vi "init.vi"(8 "error in (no error)":errorcluster, 10 "Resource":string, 11 "ScopeNi in":refnum<class "ScopeNi.lvclass">) -> (0 "error out":errorcluster, 3 "ScopeNi out":refnum<class "ScopeNi.lvclass">)   [LabVIEW 2023, in "ScopeNi.lvclass"]
doc: "Initialize the instrument by a given resource string or alias name"
uses:
  ScopeNi.lvclass
  ScopeNi.lvclass/ScopeNi.ctl
  <instrlib>/niScope/Configure/Trigger/niScope Configure Trigger Edge.vi
  Scope.lvclass
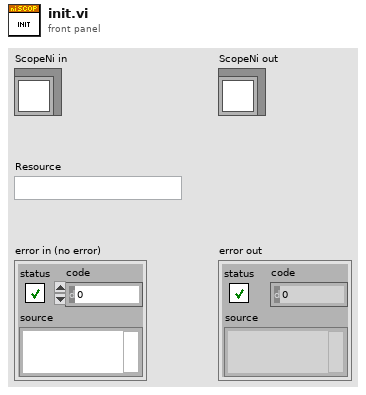
[diagram p1: front panel]
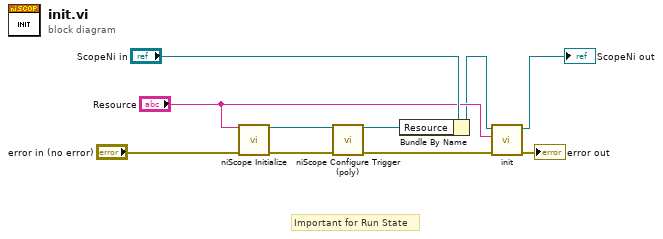
[diagram p0: block diagram]
diagram:
  # "Important for Run State"
  n1 = call <instrlib>:"niScope Initialize.vi"("resource name"="Resource", "error in"="error in (no error)") -> ("instrument handle"=w4:refnum<k15>, "error out"=w2:errorcluster)  [unwired: 12 in]
  n2 = call-poly <instrlib>:"niScope Configure Trigger (poly).vi"("instrument handle"=w4, "error in"=w2) -> ("instrument handle out"=w3:refnum<k15>, "error out"=w1:errorcluster)  [unwired: 12 in]
  n3 = Bundle By Name(cluster="ScopeNi in", "Resource"=w3) -> (w5:refnum<class "ScopeNi.lvclass">)
  n4 = call-parent "init.vi"("error in (no error)"=w1, "Resource"="Resource", "Instrument in"=w5) -> ("error out"=→"error out":errorcluster, "Instrument out"=→"ScopeNi out":refnum<class "ScopeNi.lvclass">)  [unwired: 7 in]
